vi "仪器初始化.vi"(8 "error in (no error)":errorcluster, 10 "2700":refnum<visa-resource-name>="GPIB0::16::INSTR", 11 "IT6512C":refnum<visa-resource-name>="GPIB0::16::INSTR") -> (0 "error out":errorcluster, 2 "2700":refnum<visa-resource-name>, 3 "IT6512C":refnum<visa-resource-name>)   [LabVIEW 2020]
uses:
  D/Program Files (x86)/National Instruments/LabVIEW 2020/instr.lib/IT6500/IT6500.lvlib
  D/Program Files (x86)/National Instruments/LabVIEW 2020/instr.lib/Keithley 27XX/Keithley 27XX.lvlib
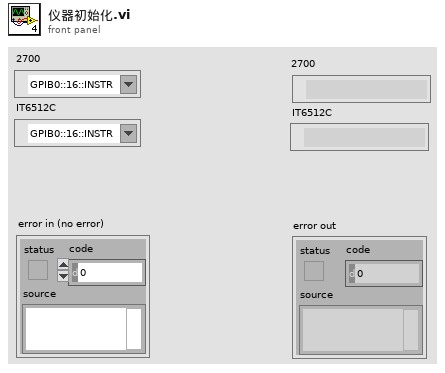
[diagram p1: front panel]
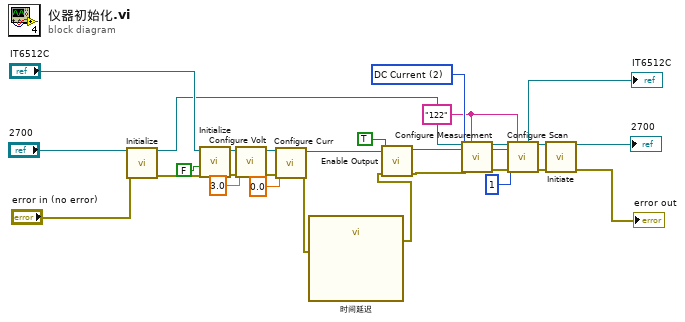
[diagram p0: block diagram]
diagram:
  w11 = u16 2 items=["DC Voltage", "AC Voltage", "DC Current", "AC Current", "Resistance", "Four-Wire Resistance", "Temperature", "Frequency", "Period", "Continuity"] ("Function (0: DC Voltage)")
  w8 = "122" ("Scan List (Empty)")
  n1 = call "Initialize.vi"("VISA resource name"="2700", "error in (no error)"="error in (no error)") -> ("VISA resource name out"=w12:refnum<visa-resource-name>, "error out"=w27:errorcluster)  [unwired: 12 in]
  n2 = call "Initialize.vi"("error in (no error)"=w27, "Reset (True)"=FALSE, "VISA resource name"="IT6512C") -> ("error out"=w23:errorcluster, "VISA resource name out"=w22:refnum<visa-resource-name>)  [unwired: 7 in]
  n3 = call "Configure Volt.vi"("error in (no error)"=w23, "Volt(0)"=3.0, "VISA resource name"=w22) -> ("error out"=w20:errorcluster, "VISA resource name out"=w19:refnum<visa-resource-name>)  [unwired: 7 in]
  n4 = call "Configure Curr.vi"("error in (no error)"=w20, "Curr(0)"=0.0, "VISA resource name"=w19) -> ("error out"=w15:errorcluster, "VISA resource name out"=w17:refnum<visa-resource-name>)  [unwired: 7 in]
  n5 = call "时间延迟"("error in (no error)"=w15) -> ("error out"=w14:errorcluster)  [unwired: 10 in]
  n6 = call "Enable Output.vi"("error in (no error)"=w14, "Enable"=TRUE, "VISA resource name"=w17) -> ("error out"=w13:errorcluster, "VISA resource name out"=→"IT6512C":refnum<visa-resource-name>)  [unwired: 7 in]
  n7 = call "Configure Measurement.vi"("VISA resource name"=w12, "Scan List (Empty)"=w8, "Function (0: DC Voltage)"=w11, "error in (no error)"=w13) -> ("VISA resource name out"=w10:refnum<visa-resource-name>, "error out"=w9:errorcluster)  [unwired: 10 in]
  n8 = call "Configure Scan.vi"("VISA resource name"=w10, "Channel List (101:110)"=w8, "Sample Count (100)"=1, "error in (no error)"=w9) -> ("VISA resource name out"=w6:refnum<visa-resource-name>, "error out"=w5:errorcluster)  [unwired: 10 in]
  n9 = call "Initiate.vi"("VISA resource name"=w6, "error in (no error)"=w5) -> ("VISA resource name out"=→"2700":refnum<visa-resource-name>, "error out"=→"error out":errorcluster)  [unwired: 12 in]
